vi "Create Filenames (SubVI).vi"(8 "error in (no error)":errorcluster, 9 "seconds since 1Jan1904":timestamp, 10 "File name":string, 11 "Session path":path) -> (0 "error out":errorcluster, 1 "binFilePath":path, 2 "topoFilePath":path, 3 "Drift File out":refnum<file>)   [LabVIEW 2014]
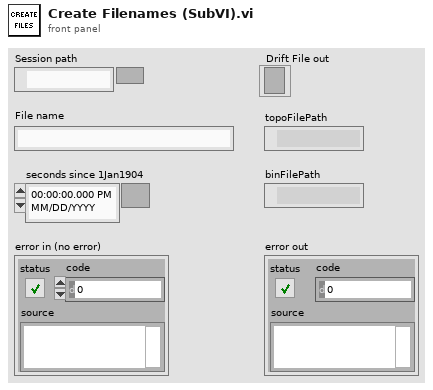
[diagram p1: front panel]
types:
  T1 = enum16{"open", "replace", "create", "open or create", "replace or create", "replace or create with confirmation"}
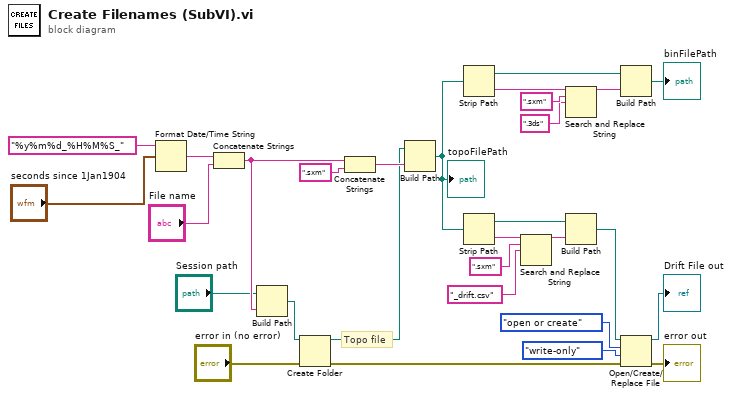
[diagram p0: block diagram]
diagram:
  # "Topo file"
  n1 = Format Date/Time String(time format string (%c)="%y%m%d_%H%M%S_", seconds (now)="seconds since 1Jan1904") -> (date/time string=w25:string)  [unwired: 1 in]
  n2 = Concatenate Strings(w25, "File name") -> (w23:string)
  n3 = Build Path(base path="Session path", name or relative path=w23) -> (appended path=w17:path)
  n4 = Create Folder(path (use dialog)=w17, error in="error in (no error)") -> (created path=w19:path, error out=w22:errorcluster)  [unwired: 1 in, 1 out]
  n5 = Concatenate Strings(w23, ".sxm" ("pattern")) -> (w20:string)
  n6 = Build Path(base path=w19, name or relative path=w20) -> (appended path=w21:path)
  "topoFilePath" <- w21
  n7 = Strip Path(path=w21) -> (stripped path=w9:path, name=w10:string)
  n8 = Strip Path(path=w21) -> (stripped path=w2:path, name=w5:string)
  n9 = Search and Replace String(input string=w5, search string=".sxm", replace string="_drift.csv" ("replace string (\"\")")) -> (result string=w4:string)  [unwired: 5 in, 3 out]
  n10 = Search and Replace String(input string=w10, search string=".sxm", replace string=".3ds" ("replace string (\"\")")) -> (result string=w8:string)  [unwired: 5 in, 3 out]
  n11 = Build Path(base path=w2, name or relative path=w4) -> (appended path=w3:path)
  n12 = Build Path(base path=w9, name or relative path=w8) -> (appended path=→"binFilePath":path)
  n13 = Open/Create/Replace File(file path (use dialog)=w3, error in=w22, operation (0:open)=T1."open or create", access (0:read/write)=enum16{"read/write", "read-only", "write-only"}."write-only") -> (refnum out=→"Drift File out":refnum<file>, error out=→"error out":errorcluster)  [unwired: 2 in, 1 out]
